vi "Compile Channel Groups.vi"(7 "Settings(JSON)":string, 8 "error in":errorcluster) -> (0 "error out":errorcluster, 3 "ChannelGroups":T1, 5 "Settings(JSON)":string)   [LabVIEW 2026, in "Template Deployment Hooks.lvlib"]
uses:
  Template Deployment Hooks.lvlib
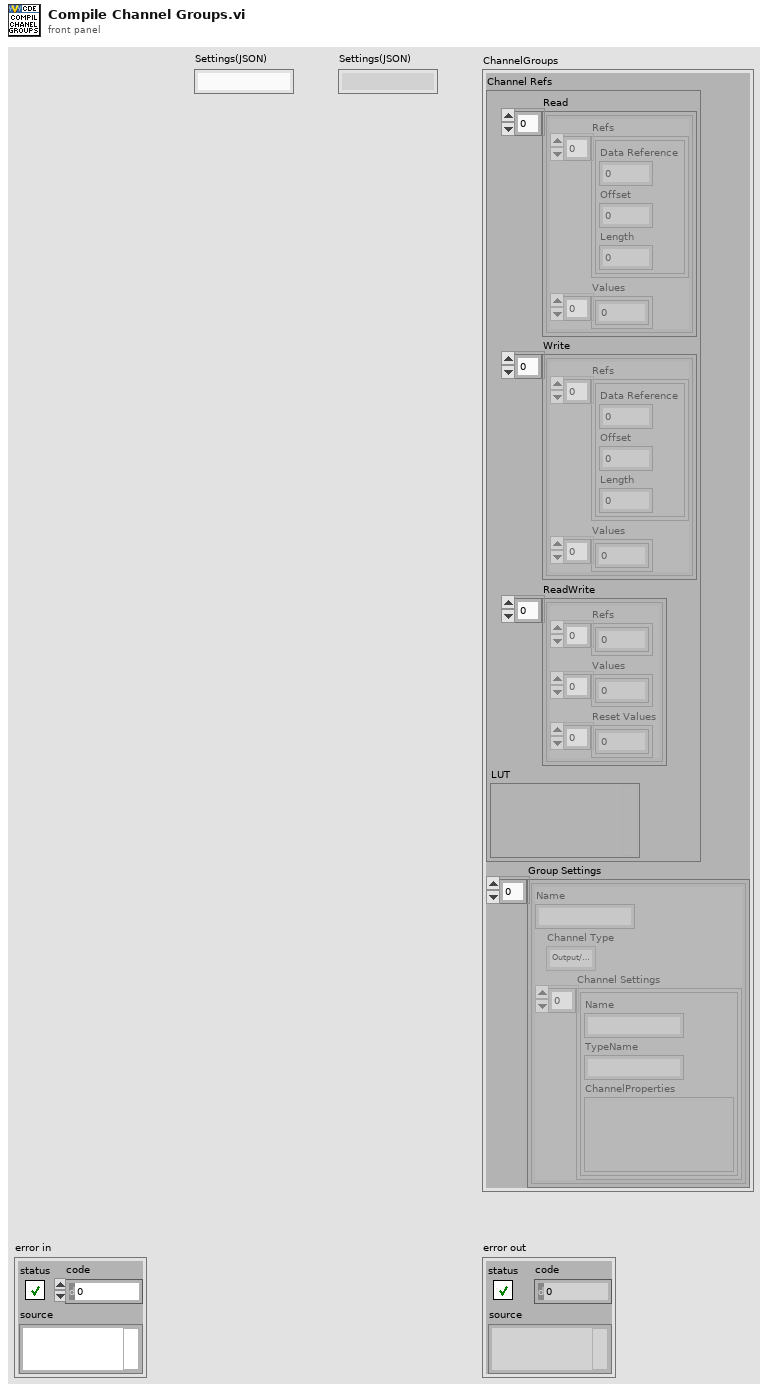
[diagram p1: front panel]
types:
  T1 = cluster{"Channel Refs":cluster{"Read":cluster{"Refs":cluster{"Data Reference":i32, "Offset":u64, "Length":u64}[], "Values":dbl[]}[], "Write":cluster{"Refs":cluster{"Data Reference":i32, "Offset":u64, "Length":u64}[], "Values":dbl[]}[], "ReadWrite":cluster{"Refs":i32[], "Values":dbl[], "Reset Values":dbl[]}[], "LUT":variant}, "Group Settings":cluster{"Name":string, "Channel Type":enum16{"Output/Write", "Input/Read", "Input/ReadWrite"}, "Channel Settings":cluster{"Name":string, "TypeName":string, "ChannelProperties":variant}[]}[]}
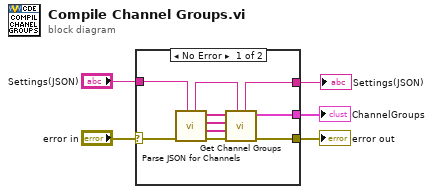
[diagram p0: block diagram]
diagram:
  n1 = case shown="No Error" "error in" {
    selector: "error in" -> [w15 w17]
    tunnel: [w14 w17] -> w5
    tunnel: "Settings(JSON)" -> [w9 w16]
    tunnel: [w12 _] -> w2
    tunnel: [w7 w16] -> w1
    frame No Error {
      n2 = call "Parse JSON for Channels.vi"("Settings(JSON)"=w9, "error in"=w15) -> ("error out"=w13:errorcluster, "Channel Paths"=w6:string[], "Channel TypeNames"=w10:string[], "Channel JSONs"=w11:string[], "Settings(JSON)"=w8:string)  [unwired: 5 in]
      n3 = call "Get Channel Groups.vi"("Settings(JSON)"=w8, "error in"=w13, "Channel Paths"=w6, "Channel TypeNames"=w10, "Channel JSONs"=w11) -> ("error out"=w14:errorcluster, "ChannelGroups"=w12:T1, "Settings(JSON)"=w7:string)  [unwired: 4 in]
    }
    frame Error {
    }
  }
  "error out" <- w5
  "ChannelGroups" <- w2
  "Settings(JSON)" <- w1
